vi "maxmin45.vi"(0 "Numeric":dbl, 2 "Numeric 2":dbl, 3 "Numeric 3":dbl, 4 "Numeric 5":dbl, 5 "Numeric 4":dbl) -> (6 "greatest":dbl, 7 "Smallest":dbl)   [LabVIEW 2014]
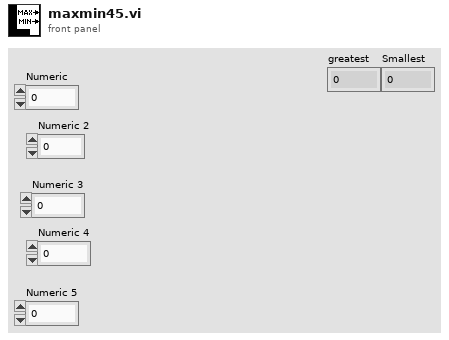
[diagram p1: front panel]
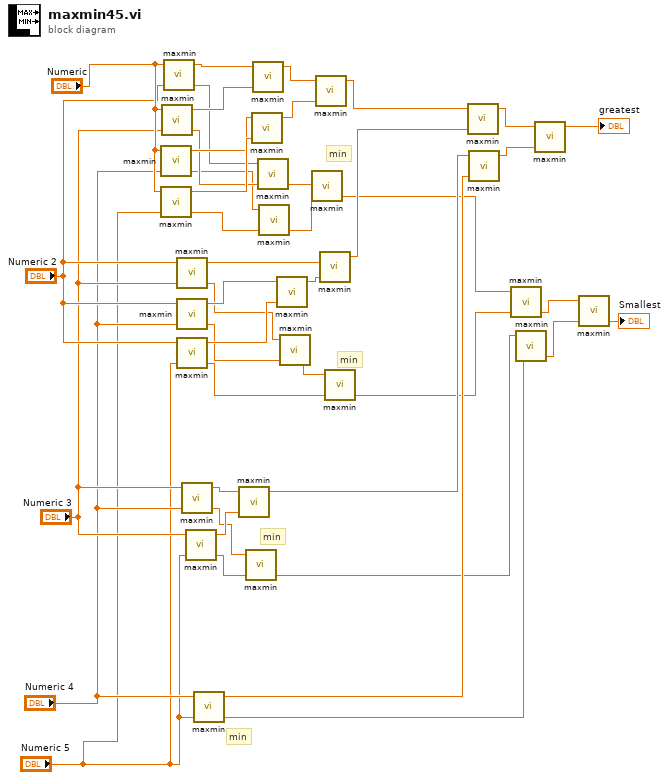
[diagram p0: block diagram]
diagram:
  # "min"
  # "min"
  # "min"
  # "min"
  n1 = call "maxmin.vi"("Numeric 2"="Numeric 4", "Numeric"="Numeric") -> ("Smallest"=w17:dbl, "greatest"=w39:dbl)  [unwired: 2 in]
  n2 = call "maxmin.vi"("Numeric 2"="Numeric 5", "Numeric"="Numeric") -> ("Smallest"=w16:dbl, "greatest"=w40:dbl)  [unwired: 2 in]
  n3 = call "maxmin.vi"("Numeric 2"="Numeric 3", "Numeric"="Numeric") -> ("Smallest"=w18:dbl, "greatest"=w41:dbl)  [unwired: 2 in]
  n4 = call "maxmin.vi"("Numeric 2"="Numeric 2", "Numeric"="Numeric") -> ("Smallest"=w19:dbl, "greatest"=w42:dbl)  [unwired: 2 in]
  n5 = call "maxmin.vi"("Numeric 2"="Numeric 3", "Numeric"="Numeric 2") -> ("Smallest"=w13:dbl, "greatest"=w34:dbl)  [unwired: 2 in]
  n6 = call "maxmin.vi"("Numeric 2"="Numeric 4", "Numeric"="Numeric 2") -> ("Smallest"=w12:dbl, "greatest"=w36:dbl)  [unwired: 2 in]
  n7 = call "maxmin.vi"("Numeric 2"="Numeric 5", "Numeric"="Numeric 2") -> ("Smallest"=w11:dbl, "greatest"=w35:dbl)  [unwired: 2 in]
  n8 = call "maxmin.vi"("Numeric 2"="Numeric 4", "Numeric"="Numeric 3") -> ("Smallest"=w9:dbl, "greatest"=w31:dbl)  [unwired: 2 in]
  n9 = call "maxmin.vi"("Numeric 2"="Numeric 5", "Numeric"="Numeric 3") -> ("Smallest"=w8:dbl, "greatest"=w30:dbl)  [unwired: 2 in]
  n10 = call "maxmin.vi"("Numeric 2"="Numeric 5", "Numeric"="Numeric 4") -> ("Smallest"=w4:dbl, "greatest"=w24:dbl)  [unwired: 2 in]
  n11 = call "maxmin.vi"("Numeric 2"=w30, "Numeric"=w31) -> ("greatest"=w25:dbl)  [unwired: 2 in, 1 out]
  n12 = call "maxmin.vi"("Numeric 2"=w8, "Numeric"=w9) -> ("Smallest"=w5:dbl)  [unwired: 2 in, 1 out]
  n13 = call "maxmin.vi"("Numeric 2"=w40, "Numeric"=w39) -> ("greatest"=w20:dbl)  [unwired: 2 in, 1 out]
  n14 = call "maxmin.vi"("Numeric 2"=w41, "Numeric"=w42) -> ("greatest"=w38:dbl)  [unwired: 2 in, 1 out]
  n15 = call "maxmin.vi"("Numeric 2"=w18, "Numeric"=w19) -> ("Smallest"=w15:dbl)  [unwired: 2 in, 1 out]
  n16 = call "maxmin.vi"("Numeric 2"=w16, "Numeric"=w17) -> ("Smallest"=w14:dbl)  [unwired: 2 in, 1 out]
  n17 = call "maxmin.vi"("Numeric 2"=w35, "Numeric"=w36) -> ("greatest"=w33:dbl)  [unwired: 2 in, 1 out]
  n18 = call "maxmin.vi"("Numeric 2"=w12, "Numeric"=w13) -> ("Smallest"=w10:dbl)  [unwired: 2 in, 1 out]
  n19 = call "maxmin.vi"("Numeric 2"=w14, "Numeric"=w15) -> ("Smallest"=w7:dbl)  [unwired: 2 in, 1 out]
  n20 = call "maxmin.vi"("Numeric 2"=w20, "Numeric"=w38) -> ("greatest"=w27:dbl)  [unwired: 2 in, 1 out]
  n21 = call "maxmin.vi"("Numeric 2"=w33, "Numeric"=w34) -> ("greatest"=w26:dbl)  [unwired: 2 in, 1 out]
  n22 = call "maxmin.vi"("Numeric 2"=w11, "Numeric"=w10) -> ("Smallest"=w6:dbl)  [unwired: 2 in, 1 out]
  n23 = call "maxmin.vi"("Numeric 2"=w26, "Numeric"=w27) -> ("greatest"=w23:dbl)  [unwired: 2 in, 1 out]
  n24 = call "maxmin.vi"("Numeric 2"=w24, "Numeric"=w25) -> ("greatest"=w22:dbl)  [unwired: 2 in, 1 out]
  n25 = call "maxmin.vi"("Numeric 2"=w6, "Numeric"=w7) -> ("Smallest"=w3:dbl)  [unwired: 2 in, 1 out]
  n26 = call "maxmin.vi"("Numeric 2"=w4, "Numeric"=w5) -> ("Smallest"=w2:dbl)  [unwired: 2 in, 1 out]
  n27 = call "maxmin.vi"("Numeric 2"=w22, "Numeric"=w23) -> ("greatest"=→"greatest":dbl)  [unwired: 2 in, 1 out]
  n28 = call "maxmin.vi"("Numeric 2"=w2, "Numeric"=w3) -> ("Smallest"=→"Smallest":dbl)  [unwired: 2 in, 1 out]
